vi "H036 Harsh Pandit SCADA Lab 2c Sem 6.vi"() -> ()   [LabVIEW 2018]
panel:
  out "Odd":bool
  out "Even":bool
  in  "Given Number":dbl
  # "Lab 2c: Develope a HMI to find whether the given number is even or odd."
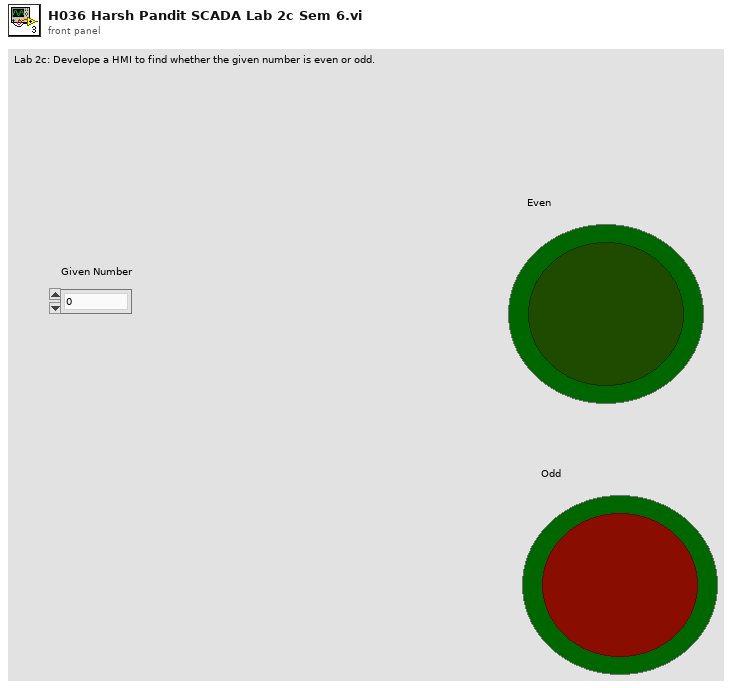
[diagram p1: front panel]
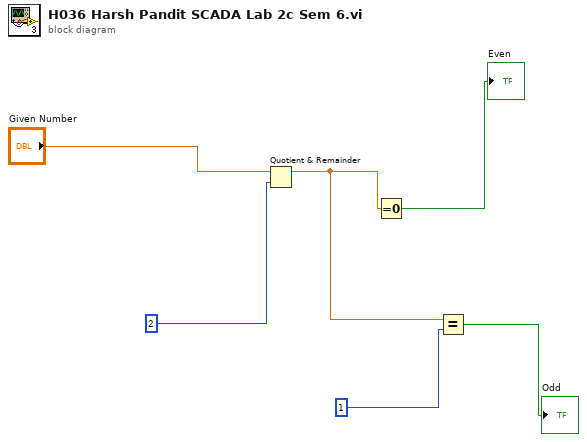
[diagram p0: block diagram]
diagram:
  n1 = Quotient & Remainder(x="Given Number", y=2) -> (x-y*floor(x/y)=w3:dbl)  [unwired: 1 out]
  n2 = Equal To 0?(x=w3) -> (x = 0?=→"Even":bool)
  n3 = Equal?(x=w3, y=1) -> (x = y?=→"Odd":bool)
